vi "generator_init.vi"(8 "error in (no error)":errorcluster, 10 "Impedance (0: 50 Ohms)":u16(ring) items=["50 Ohms", "High Impedance"], 11 "UI in":T1) -> (0 "error out":errorcluster, 3 "UI out":T1)   [LabVIEW 2017]
uses:
  ui.ctl
  classes/dc_power_supply/DC_power_supply.lvclass
  classes/report/Report.lvclass
  ui_buttons.ctl
  types/boc_type.ctl
  <instrlib>/Siglent SDG X Series/Siglent SDG X Series.lvlib
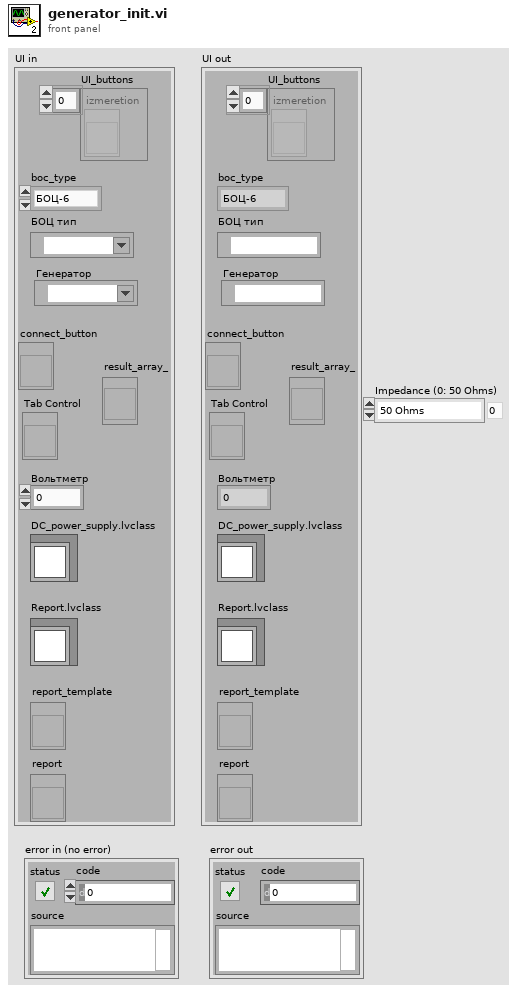
[diagram p1: front panel]
types:
  T1 = typedef "ui.ctl" = cluster{"UI_buttons":T2, "Tab Control":refnum<vi>, "connect_button":refnum<vi>, "generator":refnum<visa-resource-name>, "voltmetr":refnum<visa-resource-name>, "channel_timeout_sec":dbl, "boc_type":T3, "result_array_":refnum<vi>, "DC_power_supply.lvclass":refnum<class "DC_power_supply.lvclass">, "Report.lvclass":refnum<class "Report.lvclass">, "report_template":refnum<vi>, "report":refnum<vi>}
  T2 = typedef "ui_buttons.ctl" = refnum<vi>[]
  T3 = typedef "boc_type.ctl" = enum16{"БОЦ-6", "БОЦ-12"}
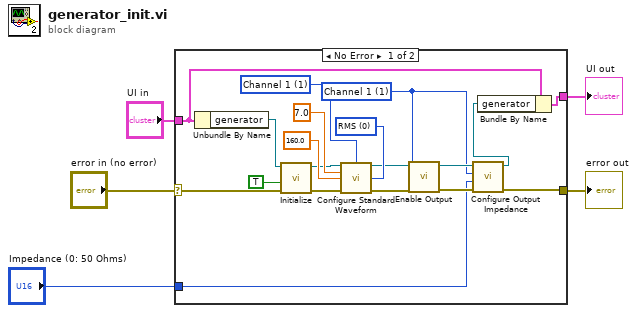
[diagram p0: block diagram]
diagram:
  n1 = case shown="No Error" "error in (no error)" {
    selector: "error in (no error)" -> [w15 w25]
    tunnel: [w24 w26] -> w5
    tunnel: "UI in" -> [w23 w26]
    tunnel: [w11 w25] -> w3
    tunnel: "Impedance (0: 50 Ohms)" -> [w6 _]
    frame No Error {
      w8 = 1 items=["Channel 1"=1, "Channel 2"=2] ("Channel (1:Channel 1)")
      w20 = 1 items=["Channel 1"=1, "Channel 2"=2] ("Channel (1:Channel 1)")
      w18 = u16 0 items=["RMS", "pp", "dBm"] ("v-type")
      n2 = Unbundle By Name(w23) -> ("generator"=w22:refnum<visa-resource-name>)
      n3 = call <instrlib>:"Initialize.vi"("error in (no error)"=w15, "Reset (True)"=TRUE, "VISA resource name"=w22) -> ("error out"=w17:errorcluster, "VISA resource name out"=w16:refnum<visa-resource-name>)  [unwired: 7 in]
      n4 = call <instrlib>:"Configure Standard Waveform.vi"("VISA resource name"=w16, "Channel (1:Channel 1)"=w20, "Amplitude (1.0 Vpp)"=7.0, "Frequency (1000 Hz)"=160.0, "v-type"=w18, "error in (no error)"=w17) -> ("VISA resource name out"=w13:refnum<visa-resource-name>, "error out"=w14:errorcluster)  [unwired: 8 in]
      n5 = call <instrlib>:"Enable Output.vi"("error in (no error)"=w14, "Channel (1:Channel 1)"=w8, "VISA resource name"=w13) -> ("error out"=w12:errorcluster, "VISA resource name out"=w10:refnum<visa-resource-name>)  [unwired: 7 in]
      n6 = call <instrlib>:"Configure Output Impedance.vi"("error in (no error)"=w12, "Impedance (0: 50 Ohms)"=w6, "Channel (1:Channel 1)"=w8, "VISA resource name"=w10) -> ("error out"=w11:errorcluster, "VISA resource name out"=w9:refnum<visa-resource-name>)  [unwired: 6 in]
      n7 = Bundle By Name(cluster=w23, "generator"=w9) -> (w24:T1)
    }
    frame Error {
    }
  }
  "UI out" <- w5
  "error out" <- w3
